vi "Configure ISIM.vi"(7 "IMPI (\"\")":string, 8 "error in (no error)":errorcluster, 9 "Enable (Off)":bool, 10 "SIM Profile Name (\"\")":string, 11 "VISA resource name":refnum<visa-resource-name>) -> (0 "error out":errorcluster, 3 "VISA resource name out":refnum<visa-resource-name>)   [LabVIEW 2015, in "Rohde&Schwarz CMXP Base.lvlib"]
doc: "The IP multimedia services identity module (ISIM) contains parameters for identifying and authenticating the DUT in the IP multimedia subsystem (IMS).\n\nAttributes:\nRSCMXPBASE_ATTR_ISIM_ENABLED\nRSCMXPBASE_ATTR_ISIM_IP_MULTIMEDIA_PRIVATE_IDENTITY\n\nRemote-control commands:\n[CONFigure:]SIMProfile:ISIM:ENABle\n[CONFigure:]SIMProfile:ISIM:IMPI"
uses:
  <instrlib>/Rohde&Schwarz CMXP Base/Rohde&Schwarz CMXP Base.lvlib
  <instrlib>/Rohde&Schwarz CMXP Base/Private/rsidr_core.llb/rsidr_core.lvlib
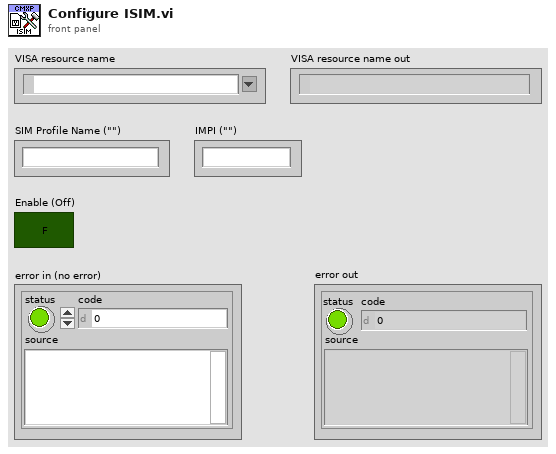
[diagram p1: front panel]
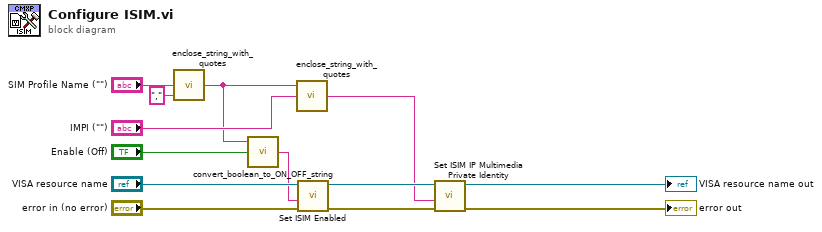
[diagram p0: block diagram]
diagram:
  n1 = call <instrlib>:"enclose_string_with_quotes.vi"("String after"=",", "String to enclose"="SIM Profile Name (\"\")") -> ("String out"=w2:string)  [unwired: 3 in]
  n2 = call <instrlib>:"convert_boolean_to_ON_OFF_string.vi"("boolean value in"="Enable (Off)", "String to add before (\"\")"=w2) -> ("string value out"=w6:string)  [unwired: 3 in]
  n3 = call <instrlib>:"enclose_string_with_quotes.vi"("String to enclose"="IMPI (\"\")", "String before"=w2) -> ("String out"=w1:string)  [unwired: 3 in]
  n4 = call "Set ISIM Enabled"("error in (no error)"="error in (no error)", "ISIM Enabled ()"=w6, "instrument handle"="VISA resource name") -> ("error out"=w11:errorcluster, "instrument handle out"=w10:refnum<visa-resource-name>)  [unwired: 7 in]
  n5 = call "Set ISIM IP Multimedia Private Identity"("error in (no error)"=w11, "ISIM IP Multimedia Private Identity ()"=w1, "instrument handle"=w10) -> ("error out"=→"error out":errorcluster, "instrument handle out"=→"VISA resource name out":refnum<visa-resource-name>)  [unwired: 7 in]
